vi "readBendingModeFile.vi"(7 "Number of Bending Mode":i32=20, 8 "error in (no error)":errorcluster, 9 "Skip Col Idx":i32[](array[numeric]), 10 "Path":path=path "/home/ttsai/Documents/stash/ts_tcs_ofc/configData/M1M3/M1M3_1um_156_force.txt", 11 "BendModeToForce in":refnum<class "BendModeToForce.lvclass">) -> (0 "error out":errorcluster, 2 "Rotation Matrix":dbl[][](array[numeric]), 3 "BendModeToForce out":refnum<class "BendModeToForce.lvclass">)   [LabVIEW 2016, in "BendModeToForce.lvclass"]
doc: "Read the mirror bending mode file. The column is the actuator forces and the row is the related bending mode."
uses:
  BendModeToForce.lvclass
  Utility/getSubArray2D.vi
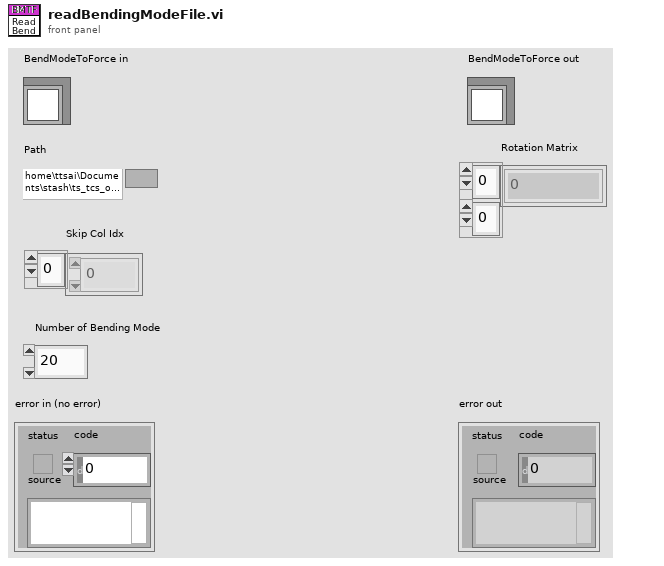
[diagram p1: front panel]
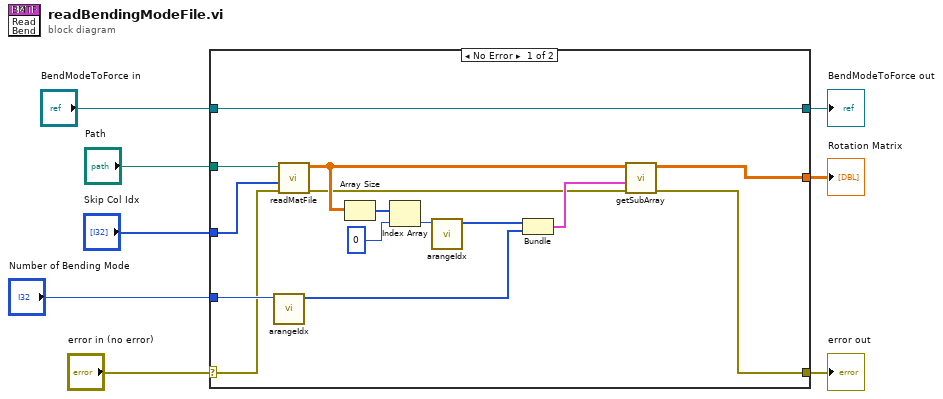
[diagram p0: block diagram]
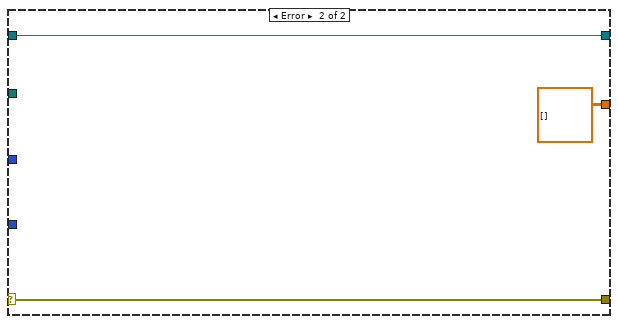
[diagram p2: hidden frame]
diagram:
  n1 = case shown="No Error" "error in (no error)" {
    selector: "error in (no error)" -> [w11 w26]
    tunnel: [w9 w26] -> w7
    tunnel: [w23 w25] -> w5
    tunnel: "BendModeToForce in" -> [w23 w25]
    tunnel: "Path" -> [w22 _]
    tunnel: "Skip Col Idx" -> [w21 _]
    tunnel: "Number of Bending Mode" -> [w17 _]
    tunnel: [w12 dbl[][] [] ("Sub-Array")] -> w1
    frame No Error {
      n2 = call "arangeIdx.vi"("Number"=w17) -> ("Idx Array"=w14:i32[])  [unwired: 10 in]
      n3 = call "readMatFile.vi"("error in (no error)"=w11, "Skip Col Idx"=w21, "Path"=w22) -> ("error out"=w10:errorcluster, "Matrix"=w16:dbl[][])  [unwired: 7 in]
      n4 = Array Size(array=w16) -> (size(s)=w20:i32[])
      n5 = Index Array(array=w20, index=0) -> (element=w19:i32)
      n6 = call "arangeIdx.vi"("Number"=w19) -> ("Idx Array"=w15:i32[])  [unwired: 10 in]
      n7 = Bundle("Idx Array"=w15, "Idx Array"=w14) -> (w13:cluster{"Idx Array":i32[], "Idx Array":i32[]})  [unwired: 1 in]
      n8 = call-poly "getSubArray.vi"("error in (no error)"=w10, "Index Array Cluster"=w13, "2D Array"=w16) -> ("error out"=w9:errorcluster, "Sub-Array"=w12:dbl[][])  [unwired: 7 in]
    }
    frame Error {
    }
  }
  "error out" <- w7
  "BendModeToForce out" <- w5
  "Rotation Matrix" <- w1
